vi "Check Ready.vi"(8 "error in (no error)":errorcluster, 11 "VISA Refnum in":refnum<visa-resource-name>) -> (0 "error out":errorcluster, 3 "VISA Refnum out":refnum<visa-resource-name>)   [LabVIEW 2012]
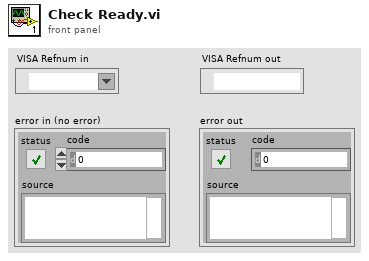
[diagram p1: front panel]
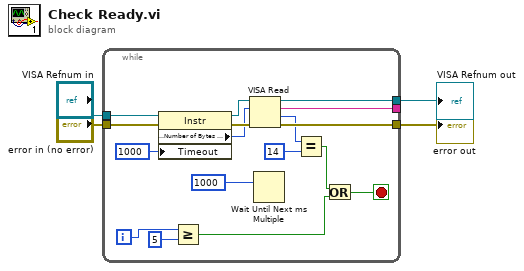
[diagram p0: block diagram]
diagram:
  n1 = while {
    tunnel: [w19] -> w4
    tunnel: [w18] -> w3
    tunnel: [w16] -> _
    tunnel: "error in (no error)" -> [w11]
    tunnel: "VISA Refnum in" -> [w12]
    i -> [w9]
    stop <- w5 stop-if-true
    n2 = property class="Instr"(reference=w12, error in=w11, "Timeout"=u32 1000 ("General Settings:Timeout Value")) -> (reference out=w20:refnum<visa-resource-name>, error out=w21:errorcluster, "Serial Settings:Number of Bytes at Serial Port"=w17:u32)
    n3 = Greater Or Equal?(x=w9, y=5) -> (x >= y?=w6:bool)
    n4 = VISA Read(VISA resource name=w20, byte count=w17, error in (no error)=w21) -> (VISA resource name out=w19:refnum<visa-resource-name>, read buffer=w16:string, return count=w14:u32, error out=w18:errorcluster)
    n5 = Wait Until Next ms Multiple(millisecond multiple=u32 1000) -> ()  [unwired: 1 out]
    n6 = Equal?(x=w14, y=u32 14) -> (x = y?=w7:bool)
    n7 = Or(x=w7, y=w6) -> (x .or. y?=w5:bool)
  }
  "VISA Refnum out" <- w4
  "error out" <- w3
